vi "Gain Add or Remove.vi"(8 "error in (no error)":errorcluster, 9 "Name Prefix":string, 10 "Size":i32, 11 "Channel Gain":T1) -> (0 "error out":errorcluster, 3 "Channel Gain out":T1)   [LabVIEW 2019, in "Instrument.DAQ.lvclass"]
uses:
  Instrument.DAQ.lvclass
  Typedefs/Channel.Gain--Cluster--Array.ctl
  Typedefs/Channel.Gain--Cluster.ctl
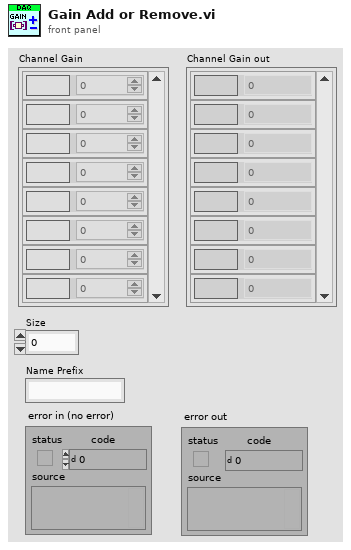
[diagram p1: front panel]
types:
  T1 = typedef "Instrument.DAQ.lvclass/Channel.Gain--Cluster--Array.ctl" = T2[]
  T2 = typedef "Instrument.DAQ.lvclass/Channel.Gain--Cluster.ctl" = cluster{"Channel":string, "Gain":dbl}
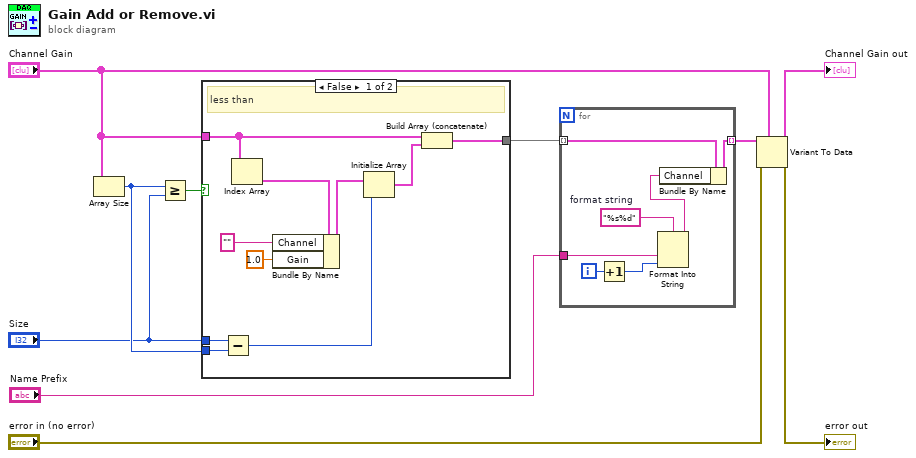
[diagram p0: block diagram]
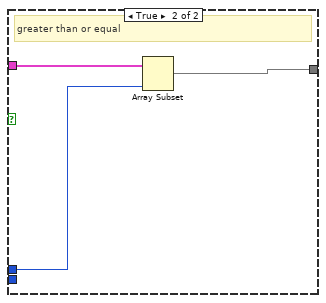
[diagram p2: hidden frame]
diagram:
  n1 = Array Size(array="Channel Gain") -> (size(s)=w10:i32)
  n2 = Greater Or Equal?(x=w10, y="Size") -> (x >= y?=w9:bool)
  n3 = case shown="False" w9 {
    tunnel: "Channel Gain" -> [w14 w23]
    tunnel: "Size" -> [w18 w22]
    tunnel: [w19 w21] -> w7
    tunnel: w10 -> [w17 _]
    frame False {
      # "less than"
      n4 = Subtract(x=w18, y=w17) -> (x-y=w16:i32)
      n5 = Index Array(array=w14) -> (element=w13:T2)  [unwired: 1 in]
      n6 = Bundle By Name(cluster=w13, "Channel"="", "Gain"=1.0) -> (w15:T2)
      n7 = Initialize Array(w15, w16) -> (w20:T2[])
      n8 = Build Array (concatenate)(w14, w20) -> (w19:T1)
    }
    frame True {
      # "greater than or equal"
      n9 = Array Subset(array=w23, length=w22) -> (w21:T1)  [unwired: 1 in]
    }
  }
  n10 = for {
    tunnel: w7 -> [w30] mode=indexing
    tunnel: [w29] -> w6 mode=indexing
    tunnel: "Name Prefix" -> [w24]
    i -> [w28]
    w27 = "%s%d"  # format string
    n11 = Increment(x=w28) -> (x+1=w25:i32)
    n12 = Format Into String(format string=w27, w24, w25) -> (resulting string=w26:string)  [unwired: 2 in, 1 out]
    n13 = Bundle By Name(cluster=w30, "Channel"=w26) -> (w29:T2)
  }
  n14 = Variant To Data(error in="error in (no error)", type="Channel Gain", Variant=w6) -> (data=→"Channel Gain out":T1, error out=→"error out":errorcluster)
